vi "SV Read Next Continuous Data.vi"(6 "reset start (F)":bool, 7 "reader ID":string="ContinuousData", 8 "error in (no error)":errorcluster, 9 "timeout (0 ms)":i32, 10 "block length (-1 = all)":i32=-1, 11 "buffer":refnum<data-value>) -> (0 "error out":errorcluster, 1 "end of buffer":bool, 2 "waveforms subset":waveform(dbl)[](array[waveform]), 3 "buffer out":refnum<data-value>)   [LabVIEW 2017]
doc: "Adds buffering to stimulus-response applications. You must manually select the polymorphic instance to use."
uses:
  <vilib>/addons/_NISVFA/_Shared subVIs/Data Objects/Waveforms (DBL)/Waveforms (N Ch).lvclass
  C:/Program Files (x86)/National Instruments/LabVIEW 2017/vi.lib/addons/_NISVFA/_Shared subVIs/Data Objects/Data/Data.lvclass
  <vilib>/addons/_NISVFA/_Shared subVIs/Data Objects/Data/Data.lvclass/Data.ctl
  <vilib>/addons/_NISVFA/_Shared subVIs/Data Objects/Waveforms (DBL)/Waveforms (N Ch).lvclass/Waveforms (N Ch).ctl
  <vilib>/addons/_NISVFA/_Shared subVIs/Data Objects/Waveforms (DBL)/Read Mode for Deleting Stale Data.vi
  <vilib>/addons/_NISVFA/_Shared subVIs/Data Objects/subVIs/Get Data Timestamp.vi
  <vilib>/addons/_NISVFA/_Shared subVIs/Common/sv_Convert Timestamp to Relative Index.vi
  <vilib>/addons/_NISVFA/_Shared subVIs/Data Objects/subVIs/Get Data Length.vi
  <vilib>/addons/_NISVFA/_Shared subVIs/Common/SV Get Data Subset.vi
  <vilib>/addons/_NISVFA/_Shared subVIs/Common/svc_Copy Waveform Subset (Index).vi
  <vilib>/addons/_NISVFA/_Shared subVIs/Common/sv_Get NI Property Name String.vi
  <vilib>/addons/_NISVFA/_Shared subVIs/Data Objects/subVIs/Get Oldest of ReaderTimestamps.vi
  <vilib>/addons/_NISVFA/_Shared subVIs/Data Objects/subVIs/Set Data Timestamp.vi
  <vilib>/addons/_NISVFA/_Shared subVIs/Data Objects/subVIs/Set Data Length.vi
  <vilib>/addons/_NISVFA/_Shared subVIs/Common/svc_Get Waveform Subset (Index).vi
  <vilib>/addons/_NISVFA/_Shared subVIs/Common/svc_Copy Array Subset (Index).vi
  <vilib>/addons/_NISVFA/_Shared subVIs/Common/svc_Get Array Subset (Index).vi
  <vilib>/addons/_NISVFA/_Shared subVIs/Common/svc_Coerce Index and Length.vi
  <vilib>/addons/_NISVFA/_Shared subVIs/Common/svc_Conditional Merge Error.vi
  <vilib>/Utility/error.llb/Trim Whitespace.vi
  <vilib>/addons/_NISVFA/_Shared subVIs/Data Objects/Data/Data.lvclass
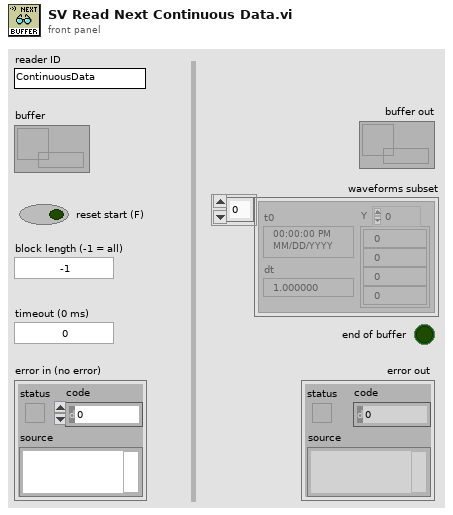
[diagram p1: front panel]
types:
  T1 = enum16{"Data Ready", "First Sample Not Yet Available", "Last Sample Not Yet Available", "Data No Longer Available"}
  T2 = typedef "svc_Delete Data Options (enum).ctl" = enum16{"Write", "Read", "Release"}
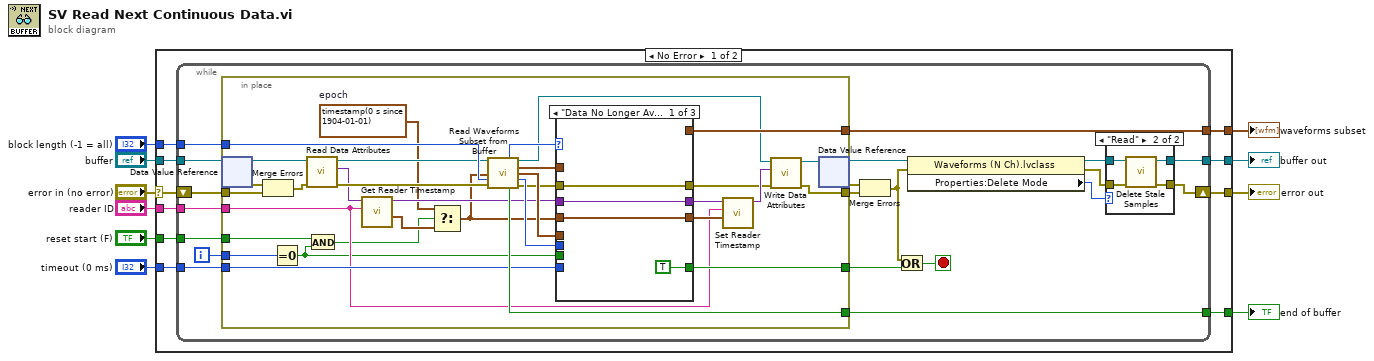
[diagram p0: block diagram]
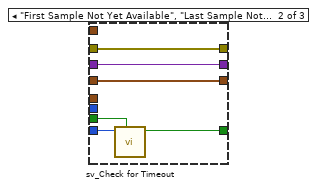
[diagram p3: hidden frame]
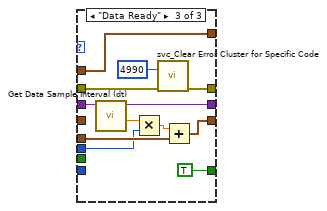
[diagram p4: hidden frame]
diagram:
  n1 = case shown="No Error" "error in (no error)" {
    selector: "error in (no error)" -> [w14 w103]
    tunnel: [w12 w102] -> w10
    tunnel: [w13 w103] -> w9
    tunnel: "block length (-1 = all)" -> [w20 _]
    tunnel: [w19 _] -> w7
    tunnel: "buffer" -> [w15 w102]
    tunnel: [w18 _] -> w5
    tunnel: "reset start (F)" -> [w17 _]
    tunnel: "reader ID" -> [w16 _]
    tunnel: "timeout (0 ms)" -> [w11 _]
    frame No Error {
      n2 = while {
        tunnel: w20 -> [w40]
        tunnel: [w39] -> w19
        tunnel: [w38] -> w18
        tunnel: w17 -> [w37]
        tunnel: w16 -> [w36]
        tunnel: w15 -> [w35]
        tunnel: [w25] -> w12
        shift-right: [w24] -> w13
        shift-left: w14 -> [w34]
        tunnel: w11 -> [w30]
        i -> [w31]
        stop <- w21 stop-if-true
        n3 = in-place {
          in-place-border: [w52] -> w33
          in-place-border: w40 -> [w79]
          in-place-border: [w76] -> w39
          in-place-border: [w73] -> w38
          in-place-border: w34 -> [w64]
          in-place-border: w37 -> [w49]
          in-place-border: w36 -> [w51]
          in-place-border: w31 -> [w50]
          in-place-border: w30 -> [w61]
          in-place-border: [w60] -> w22
          w67 = timestamp(0 s since 1904-01-01)  # epoch
          n4 = in-place-dvr #1(w35) -> (w65:refnum<class "Waveforms (N Ch).lvclass">, w63:errorcluster)
          n5 = Merge Errors(w63, w64) -> (w62:errorcluster)
          n6 = Equal To 0?(x=w50) -> (x = 0?=w47:bool)
          n7 = call <vilib>:"Read Data Attributes.vi"("error in (no error)"=w62, "Data in"=w65) -> ("error out"=w70:errorcluster, "data attributes"=w69:variant, "Data out"=w75:refnum<class "Waveforms (N Ch).lvclass">)  [unwired: 7 in]
          n8 = And(x=w49, y=w47) -> (x .and. y?=w48:bool)
          n9 = call <vilib>:"Get Reader Timestamp.vi"("ID"=w51, "data attributes"=w69) -> ("timestamp"=w66:timestamp, "data attributes"=w68:variant)  [unwired: 8 in]
          n10 = Select(t=w67, s=w48, f=w66) -> (s? t:f=w56:timestamp)
          n11 = call <vilib>:"Read Waveforms Subset from Buffer.vi"("Waveforms (N Ch)"=w75, "timestamp"=w56, "block length"=w79, "error in (no error)"=w70) -> ("subset status"=w71:T1, "Waveforms (N Ch)"=w54:refnum<class "Waveforms (N Ch).lvclass">, "waveforms subset"=w74:waveform(dbl)[], "actual timestamp"=w78:timestamp, "actual length"=w77:i32, "end of buffer"=w76:bool, "error out"=w72:errorcluster)  [unwired: 5 in]
          n12 = case shown="\"Data No Longer Available\", Default" w71 {
            tunnel: [w83 w89 w92] -> w55
            tunnel: w78 -> [_ _ w101]
            tunnel: w77 -> [_ _ w100]
            tunnel: w68 -> [w80 w86 w97]
            tunnel: w74 -> [_ _ w96]
            tunnel: [_ _ w96] -> w73
            tunnel: w72 -> [w83 w89 w94]
            tunnel: w61 -> [_ w88 _]
            tunnel: [TRUE ("timeout") w87 TRUE ("timeout")] -> w60
            tunnel: [w81 w85 w91] -> w58
            tunnel: [w80 w86 w90] -> w57
            tunnel: w56 -> [w81 w85 _]
            tunnel: w47 -> [_ w84 _]
            frame "Data No Longer Available", Default {
            }
            frame "First Sample Not Yet Available", "Last Sample Not Yet Available" {
              n13 = call <vilib>:"sv_Check for Timeout.vi"("reset"=w84, "timeout [ms]"=w88) -> ("timeout"=w87:bool)  [unwired: 8 in, 1 out]
            }
            frame "Data Ready" {
              n14 = call <vilib>:"Get Data Sample Interval (dt).vi"("variant in"=w97) -> ("dt [s]"=w98:dbl, "variant out"=w90:variant)  [unwired: 9 in]
              n15 = Multiply(x=w98, y=w100) -> (x*y=w99:dbl)
              n16 = call <vilib>:"svc_Clear Error Cluster for Specific Code.vi"("error in (no error)"=w94, "code"=4990) -> ("error out"=w92:errorcluster)  [unwired: 12 in, 1 out]
              n17 = Add(x=w99, y=w101) -> (x+y=w91:timestamp)
            }
          }
          n18 = call <vilib>:"Set Reader Timestamp.vi"("timestamp"=w58, "ID"=w51, "data attributes in"=w57) -> ("data attributes out"=w59:variant)  [unwired: 8 in]
          n19 = call <vilib>:"Write Data Attributes.vi"("error in (no error)"=w55, "data attributes"=w59, "Data in"=w54) -> ("error out"=w52:errorcluster, "Data out"=w53:refnum<class "Waveforms (N Ch).lvclass">)  [unwired: 7 in]
          n20 = in-place-dvr #1(w53) -> (w26:refnum<data-value>, w32:errorcluster)
        }
        n21 = Merge Errors(w32, w33) -> (w23:errorcluster)
        n22 = Or(x=w23, y=w22) -> (x .or. y?=w21:bool)
        n23 = property class="Waveforms (N Ch).lvclass"(reference=w26, error in=w23) -> (reference out=w28:refnum<data-value>, error out=w27:errorcluster, "Properties:Delete Mode"=w29:T2)
        n24 = case shown="\"Read\"" w29 {
          tunnel: [w42 w45] -> w25
          tunnel: w28 -> [w42 w46]
          tunnel: w27 -> [w41 w44]
          tunnel: [w41 w43] -> w24
          frame Default {
          }
          frame "Read" {
            n25 = call <vilib>:"Delete Stale Samples.vi"("error in (no error)"=w44, "buffer"=w46) -> ("error out"=w43:errorcluster, "buffer"=w45:refnum<data-value>)  [unwired: 6 in, 2 out]
          }
        }
      }
    }
    frame Error {
    }
  }
  "buffer out" <- w10
  "error out" <- w9
  "waveforms subset" <- w5
  "end of buffer" <- w7
